vi "WhiteScreenTest_Startup.vi"() -> (0 "ErrorOut":errorcluster)   [LabVIEW 2018] (continued)
-51.99405193395278, -67.01264267414084, -53.44571979526376, -57.99170790064061, -81.70961030405843, -57.55954298568111, -65.02167716156492, -63.670039415871095, -66.27707836992371, -72.55910236513691, -72.7711109939143, -62.13879248220557, -81.54101193978573, -58.629597809474696, -56.28921520683527, -62.01138186186228, -61.61803085838006, -67.34927370509035, -71.65909904633395, -51.41437767083715, -80.31871825611697, -68.62589077386892, -56.503103976004134, -68.56520281728666, -68.07660380418503, -66.43496315022747, -80.55706592055753, -58.34547433203358, -80.86357761750227, -67.11611209017593, -67.39506376816462, -61.3536075715084, -57.86340014748689, -63.774368883554196, -65.72800124970155, -52.20213098851085, -59.70633504561058, -84.09135578340957, -93.10187122260785, -115.8843421262331, -59.4590004904725, -54.15581280534354, -64.41974754094588, -65.11772802657723, -59.72007368025384, -54.860367458875366, -64.71599198424335, -88.15700585273521, -67.79336517822267, -53.60791978937983, -63.288608307220095, -58.97631404304433, -56.56722195249055, -56.08704954963907, -53.87328284835936, -54.328629340092355, -55.41015013610399, -66.24988345447511, -63.81115391904144, -59.56325497844647, -56.94831717827518, -61.65160219622933, -64.17056469987938, -77.14151841475712, -65.6193156486078, -58.86248673523286, -60.1165495622408, -63.36871733225281, -60.84953671101233, -74.8582840465121, -59.88998847841493, -95.93625941689842, -59.88299394657023, -58.812327143828576, -60.07365977395545, -60.65812972265841, -55.29460982336834, -54.39350693136425, -64.44221359336854, -56.66420968725436, -57.849249090192934, -58.12466513592309, -57.45583386749336, -54.61500881558725, -61.345460649574996, -58.25358949545251, -54.81079112114542, -69.31075240072312, -75.37140100124691, -80.95747396257286, -65.41178936486318, -52.611019655802245, -65.58758224223078, -63.071696702033954, -108.10508856206985, -60.231868757101445, -73.66935735300541, -54.45286974455788, -65.5685924636773, -67.99482155268655, -61.14400427511112, -58.82484247502318, -60.60898321122287, -59.39233587194578, -63.81115391904144, -61.2240798652709, -73.46555302607382, -62.66606303410514, -59.16259174067152, -64.56672625582956, -56.53264364522695, -57.97450072113913, -57.74797307623616, -69.70157942586468, -66.1016740458054, -78.55011000645786, -69.9180460463688, -57.80973682485905, -52.29836944058602, -65.19040261658174, -54.23115847512327, -70.88024189200894, -52.42606516970066, -88.9193056485365, -84.95782085255706, -53.597020716062, -59.4256102722857, -58.68806374826783, -69.35757045363206, -51.922125139306594, -62.54072323990115, -69.50894243068942, -84.004540711267, -70.72744912841324, -64.00259486210794, -60.377994964097574, -70.54512838063863, -53.717597051139585, -55.80413177641689, -55.66574153199439, -61.19196937503859, -70.21106198010139, -71.59962582422565, -54.769672326943116, -66.36599807965678, -82.71277721205894, -52.74962062202692, -61.4436833506844, -85.00566633827245, -86.4525103194963, -70.3349775889819, -71.30766780674031, -64.72757074243842, -59.04654597071872, -63.24880327085554, -65.72800124970155, -49.792492705188714, -65.00973814322239, -51.33087211577806, -80.23084283247556, -54.61097220706987, -60.876641068095076, -67.42571235653492, -65.09362499882167, -58.53496442470185, -60.58262362643337, -96.55537745017114, -56.98701428601347, -53.28797453185026, -82.1980867315271, -59.027340759098955, -79.26102778332853, -65.3435997401024, -78.11942920258147, -64.15418040896233, -66.17549252828113, -52.62905623918589, -61.42724290107348, -77.7072560203516, -64.62386162425068, -57.423315192286346, -77.09935131389628, -60.27183207943016, -75.62058384231338, -57.708874914398926, -56.58703708992575, -62.92176524070543, -52.13798445576547, -58.60202729712321, -72.01150979498112, -59.50930474837666, -75.2665584276316, -70.90226945622248, -56.44429612900094, -51.53222748846188, -55.38386792788341, -64.08892165389514, -58.14797741957073, -90.74071668652113, -84.22306952305414, -59.67207429490822, -52.276196407765845, -68.53069558583377, -68.44496668642603, -58.11884590614199, -62.16093188737036, -62.62410087728153, -68.44496668642603, -58.39025269247278, -59.94612909219138, -73.32258465708762, -57.55954298568111, -53.4833218966046, -55.42771169707262, -65.04559986722944, -65.02167716156492, -64.87938036213663, -52.1099574921515, -59.95669213234839, -53.6662582435933, -67.198199716695, -55.663489389713824, -75.93213175750054, -66.78742748371917, -65.41178936486318, -58.20650719235265, -65.0815961571202, -78.00314899099467, -84.40154908991724, -54.75327403235176, -83.83323258754874, -74.69316809415548, -64.46473238305185, -69.01640908021349, -50.83910224754056, -60.7380559933847, -51.59980479701239, -55.42331829191223, -63.43936573152218, -61.32918753286523, -115.8843421262331, -58.48044138560088, -71.73095706023176, -72.63805754335351, -61.30888487978432, -56.00736133181352, -52.9460711732055, -62.294852163718495, -59.83417450278508, -52.545716476460804, -87.0271131916835, -56.06589110459543, -92.66575066808954, -78.74791082859372, -68.80143089608728, -53.00904327904521, -63.74817995109995, -70.04829243356986, -65.54964020199756, -61.12011136114078, -83.0197794113686, -66.44881586021592, -68.03562552743497, -60.98583086480918, -67.75357665166754, -62.79306219219861, -57.38282125288405, -61.47664901886427, -59.17232588661076, -65.31276396941814, -72.97421667524495, -60.27183207943016, -64.35823581751049, -51.88560352159029, -62.698827642682254, -58.31870730180095, -59.114068622547016, -80.1437650787519, -76.74822277376467, -65.02167716156492, -61.349533245687944, -59.1237536309416, -74.89165103667418, -62.21873461150245, -49.9438768204733, -55.64773918094529, -57.1591608304284, -50.85955205276931, -78.11942920258147, -68.8458224607262, -75.2665584276316, -71.68299196030429, -51.86133279390611, -61.59710827647664, -84.26737907065356, -64.36381152240443, -74.62790933908832, -57.46126437995087, -96.55537745017114, -71.37693164554997, -110.5159478725686, -76.87068826675005, -62.77414108152802, -60.81480040268996, -69.58553365591192, -53.578883066491635, -55.38824329854079, -66.51838106716721, -52.92573624243261, -60.08079476870609, -53.76182148597548, -60.989753580055, -82.34234508908514, -58.86248673523286, -67.13843005293714, -63.14509415266779, -70.78173902996198, -62.984354672270875, -61.98523100514074, -53.52467497348035, -64.19793419062762, -63.35866704322458, -59.322833066623296, -66.06164756214434, -65.43047096765142, -59.702903459095715, -54.41918572771261, -55.069738493302985, -88.0246865135197, -63.10098832784568, -51.225375139342894, -68.70448657082216, -55.57383453153566, -63.01338041302321, -59.41894615253175, -51.391268957464284, -80.0574706437699, -76.97395083542065, -57.65329538465085, -73.29424490235556, -59.43895241630013, -61.534612941440336, -73.07049131842601, -55.25352624879768, -73.96822887751696, -56.56474793571346, -69.64338106738398, -65.14189176731313, -71.87630832579441, -71.45837664659064, -49.74741788735506, -94.03851706113451, -58.806075595871924, -68.58250309248953, -82.78861159907069, -66.70876658826313, -68.462051285777, -57.05966921811025, -59.45565623385853, -53.25463195735258, -73.98341969620992, -70.82539325774144, -71.49349444053763, -69.13489894768142, -60.47790367814803, -59.15286746208921, -69.45189766398155, -62.727000937528324, -84.3118942317391, -56.6367547446168, -75.23186399560109, -52.1660935431082, -60.907711540600666, -56.26760663806902, -74.33961719286634, -65.93598771642783, -62.10788290425561, -74.33961719286634, -57.7647783360084, -54.58276340707521, -78.9754234684336, -80.52694658655275, -73.43678838683073, -75.67483280875109, -58.58369087867003, -64.79733832268226, -84.8628398786199, -61.85553547398538, -62.797798306834416, -49.456535410939274, -74.32385219342672, -54.37970830574462, -63.096100174873676, -56.06354304437077, -95.64106689530826, -70.88024189200894, -68.58250309248953, -78.45271830700355, -64.36381152240443, -78.16633883150865, -58.73757611624553, -67.97042221778648, -58.12175507978066, -57.321060647676155, -59.3459447625382, -59.11084245806395, -55.9144501939028, -72.93325006494365, -67.13843005293714, -63.135275318647835, -72.24962391387751, -59.28005851453177, -65.13584512355794, -66.50442761016166, -56.935452753657195, -70.55575774460704, -63.14018347940979, -64.94433782793823, -85.7535514055914, -69.52803298425346, -51.88864168471941, -64.22538199189958, -94.67404741663125, -58.07820983932687, -61.501447826297984, -72.40311518841392, -65.9031911032867, -65.74086912554111, -70.75998618617399, -58.743783169195815, -72.33886176668707, -68.57384905491571, -56.231700170696165, -76.95320920571854, -66.3043505986688, -55.827010394463606, -59.37242649088039, -61.47664901886427, -54.75327403235176, -57.20929627668493, -57.75357155903293, -64.70442718477156, -70.66270422572774, -59.448971216166406, -69.64338106738398, -62.35799390554727, -61.345460649574996, -60.17043287185472, -63.78486450823356, -81.24480659023706, -57.16705955462927, -62.085865451395556, -59.542988069499735, -59.23420591784562, -67.47958413870552, -57.64221801621441, -61.702180520776785, -65.52442862375423, -74.41883316736389, -66.1016740458054, -68.3093743230275, -72.79794457784413, -83.66493002506755, -62.78359697189443, -62.727000937528324, -62.79306219219861, -69.97794010149332, -106.18005458050143, -91.09605360575071, -80.0574706437699, -90.5678651632339, -84.17896369823202, -63.27366205646876, -70.90226945622248, -93.44248688497498, -61.71486687924905, -61.484908167028344, -86.4525103194963, -62.10347536914477, -65.84443828268391, -69.64338106738398, -92.55974958955161, -60.93108061427673, -61.88994986066991, -70.97976670400445, -72.63805754335351, -59.188571445108, -59.027340759098955, -90.23123413228441, -67.28855831253992, -61.52216258278157, -60.268192162862114, -70.7382825570067, -63.36871733225281, -56.32533800588815, -78.94987618302852, -75.11141218888855, -70.64121933432824, -62.916967541180576, -56.0494667395707, -61.72333378182871, -59.322833066623296, -59.130215739639986, -73.84756061980656, -64.70442718477156, -63.51053828904819, -65.09964508060068, -85.29786151567325, -56.38827489577944, -89.43797250218225, -73.3795165749292, -70.20080756971822, -64.09976733057331, -67.25834411433442, -67.4333898279331, -66.46268860305295, -71.37693164554997, -48.24420036050936, -68.10951292736854, -72.12356428124627, -52.92065923781558, -62.43979165363363, -65.06958237972034, -62.394262379750494, -72.63805754335351, -65.03363105719274, -72.35167806785861, -65.27589140640507, -55.767639102832625, -70.01807823536436, -70.82539325774144, -67.5804415173883, -65.72157377877431, -60.084364257119354, -69.7601330155891, -58.83110626891206, -108.65340922603647, -67.00529453130741, -60.876641068095076, -59.542988069499735, -63.75864694613728, -80.64799551131347, -58.30683477553303, -75.65671571177037, -83.45862099838286, -57.35860668386382, -56.33016467265663, -71.238900487172, -91.0059778265747, -68.86363676482424, -60.715151883817335, -76.29274197049554, -69.26416173119159, -71.10282728369415, -62.54072323990115, -71.63526549370167, -65.67670166221052, -72.61166688021697, -56.56474793571346, -87.95920503059935, -60.006140695445445, -59.4590004904725, -54.250573579908725, -59.80638882079618, -63.449500967541546, -64.64106880375215, -75.02629184336465, -72.71766795875487, -73.09817676332747, -66.84504327252878, -82.5257732396841, -57.87757211047214, -53.427865704868985, -62.35346997242876, -58.0003230785883, -56.33982529784368, -70.63049490615708, -82.16235857104732, -60.80324952832628, -64.9088519674983, -70.01807823536436, -77.75218818680568, -57.58152008578582, -61.26436971869881, -55.120674896161084, -60.5901475483877, -83.83323258754874, -59.472389187691185, -64.54396705179721, -69.19008414301271, -66.16202866642189, -62.52229287880461, -66.24309675451039, -88.15700585273521, -76.44872914721853, -75.87641233657254, -71.03550770917977, -64.15418040896233, -56.81282418633612, -56.76471348763396, -79.26102778332853, -65.02167716156492, -57.05966921811025, -68.6345919082523, -78.77292518435783, -80.80148678584987, -71.19332795490877, -60.41118238908704, -63.30857293461339, -60.21375850063715, -69.03454330111458, -63.790116629908674, -55.538205892623374, -66.25667495918356, -76.56740694948036, -73.05667850106471, -58.36634489193626, -60.07365977395545, -57.59528138494674, -70.20080756971822, -66.02178739399196, -78.72296152974505, -52.49055616889071, -57.614580428673754, -54.21178258487631, -63.08145064288444, -81.88122489871265, -60.96232819890859, -84.26737907065356, -77.18387168443718, -59.104393382190814, -58.209443076078706, -75.78425985079298, -83.17704522854666, -72.93325006494365, -55.656736133539106, -73.62531902011878, -56.77988028921224, -62.02011467994374, -68.38540906718583, -67.05685012564672, -59.22767340142021, -56.50556214385872, -63.32857919838175, -74.01387369004044, -95.07660997858827, -58.18012459360005, -64.13237812685045, -60.41857299037708, -63.98649471846863, -78.3084599494455, -88.9917059921967, -53.82854277503649, -53.27743277254765, -52.8599438452651, -66.94671114313334, -55.39700003123463, -72.08606716510013, -54.225341597734335, -67.7853942596087, -71.10282728369415, -59.98138455267408, -82.5628835374147, -55.95150673442901, -68.82804117667325, -54.39942670939845, -79.8310766559049, -56.953467782425754, -72.19900110510912, -60.253646291993284, -61.11216026246759, -73.18171575279334, -59.56663696332196, -56.38827489577944, -63.05221852275313, -71.03550770917977, -79.91534952583305, -65.98869664024195, -73.46555302607382, -74.5954456871255, -58.4412554709403, -77.91112910075469, -59.00179347369386, -85.15065146578425, -57.1119045772306, -71.97444728912444, -111.99471534415147, -72.17378952686579, -70.54512838063863, -66.18897531335372, -68.20892314340054, -66.04169677505735, -70.1701099435229, -103.86658696945702, -62.764694502724275, -68.54793368571038, -61.567893113587196, -68.97122293920182, -67.44107344868831, -67.18322235221623, -59.04654597071872, -63.24880327085554, -58.08400446348373, -72.53292772406871, -68.56520281728666, -61.18796311062453, -66.16875823527027, -85.9632428146347, -72.66452100841161, -63.99185843121669, -76.8092600952713, -65.80546869625675, -63.530970671639516, -69.87832342232358, -82.9421028736071, -66.1016740458054, -99.10426791904789, -73.81762923826997, -72.27503584926745, -58.32167773068364, -71.47006829946992, -68.42791245971216, -66.881229660213, -76.44872914721853, -81.57449539437292, -75.78425985079298, -72.65128015054688, -72.94688617242807, -75.58458755242262, -61.31700078551376, -55.772193102443445, -67.3188679744054, -62.5591890781343, -61.702180520776785, -71.13666506128303, -71.49349444053763, -72.08606716510013, -97.39007758963268, -67.80134272545996, -75.44193808375724, -66.8739814543525, -63.863949869585916, -66.40041864044619, -60.593911723440904, -85.00566633827245, -68.20892314340054, -71.40013117318102, -71.70694453204936, -84.3118942317391, -64.08350341031704, -73.3795165749292, -68.66947558305529, -64.90295039856406, -76.44872914721853, -64.87938036213663, -67.36451278692888, -76.2156893474037, -71.803357403892, -80.23084283247556, -68.66947558305529, -81.95073969565235, -72.50682430660166, -74.66048322437624, -65.04559986722944, -74.05973672560452, -72.66452100841161, -74.29239970623465, -72.49379918579547, -59.66181988452505, -69.47087492041769, -84.49204976113185, -67.52600197120663, -66.95401453138103, -79.42047189702586, -63.94369263965309, -83.66493002506755, -88.56528023385471, -78.92439675237901, -77.3768100315248, -88.56528023385471, -79.42047189702586, -82.05596561359027, -78.16633883150865, -75.54872582841557, -77.14151841475712, -77.77473343807586, -73.87758568344123, -66.04169677505735, -83.54061295051198, -74.57925496598259, -78.4769736928713, -70.69502205528289, -78.11942920258147, -65.03363105719274, -70.70581890504388, -82.78861159907069, -71.99913970945016, -70.74912823368484, -80.1437650787519, -71.92525230951662, -77.3984891367964, -74.02913701863835, -70.66270422572774, -70.53451078132562, -81.44125714141563, -77.5296027951205, -90.39807312011936, -70.09886187065311, -72.12356428124627, -92.45490701593633, -88.70532651670183, -68.49631203647937, -97.21722606634546, -104.95374904760712, -75.35384747393371, -75.60256881354482, -97.21722606634546, -79.20846326824847, -96.3968118565532, -72.3773621528131, -81.37532561040814, -71.02433356697281, -81.30984412748779, -67.42571235653492, -78.35630543516089, -81.40823473359166, -85.70183699463703, -71.803357403892, -89.21224444052623, -93.32759928426387, -89.13816685234738, -78.18987994761696, -96.88059503539597, -77.84268885802032, -108.65340922603647, -95.35468741981339, -71.82761278975974, -75.83944504612427, -103.86658696945702, -85.24854007026573, -79.97194556019917, -80.37775228857197, -90.74071668652113, -88.63504781409856, -73.02911239014207, -83.25665564394805, -89.90601654705961, -75.11141218888855, -100.20812799967334, -85.49772291133223, -71.25032752842785, -78.89898481698907, -89.74745095344164, -78.35630543516089, -76.2156893474037, -80.31871825611697, -76.62730100460487, -84.35661692346315, -86.1235752376158, -85.24854007026573, -86.90940619345022, -105.75362882215944, -102.58562032000998, -88.9193056485365, -81.50764494962365, -84.26737907065356, -80.55706592055753, -85.91038868644006, -79.85908543492619, -86.177620450987, -87.57543385565012, -77.57370861994258, -93.79564332914123, -100.93706080531254, -107.5864217084241, -76.48812550649035, -85.19947090956941, -96.24082467983021, -83.0197794113686, -86.67823838115231, -82.0912989868688, -72.81138956953345, -89.59146377671865, -79.05247609152548, -86.9680791592285, -89.59146377671865, -111.22686564943922, -95.35468741981339, -77.77473343807586, -84.004540711267, -82.34234508908514, -96.55537745017114, -80.92607295253859, -110.5159478725686, -75.80261966500962, -78.5991791671542, -85.19947090956941, -84.004540711267, -84.81569973462018, -86.90940619345022, -84.35661692346315, -81.30984412748779, -82.60013795316792, -95.78752775545891, -117.16530877568013, -84.768790105693, -84.72210874836932, -76.2156893474037, -91.37146965148088, -88.9917059921967, -108.10508856206985, -90.23123413228441, -89.43797250218225, -82.26994474542494, -86.79312598186345, -82.78861159907069, -108.65340922603647, -87.89416749334862, -87.08651276227181, -97.92814384321613, -86.4525103194963, -95.93625941689842, -80.55706592055753, -79.80314941638477, -95.07660997858827, -90.39807312011936, -95.93625941689842, -90.14889027905289, -105.34535444103992, -112.82941548361299, -87.26695068374008, -90.91673997376512, -91.75144011322664, -92.45490701593633, -85.85782417136002, -102.89018558294177, -95.93625941689842, -107.5864217084241, -102.29042779841981, -90.23123413228441, -82.26994474542494, -91.27878294010458, -82.71277721205894, -118.64407624726303, -82.23394845553418, -91.9472224187848, -89.43797250218225, -82.67508364686299, -109.23498122312157, -86.62130646331073, -98.89795889236316, -106.18005458050143, -86.79312598186345, -87.82956792263298, -99.3151115712011, -87.70165936100221, -99.10426791904789, -89.51441115362678, -112.82941548361299, -93.55876709656178, -115.8843421262331, -87.26695068374008, -87.51293852061383, -84.62942203699302, -94.54352839646018, -87.38915615802296, -88.0246865135197, -103.86658696945702, -94.28769990220098, -92.2485979892516, -93.79564332914123, -110.5159478725686, -88.42724907547671, -83.05885482181219, -87.14628242602967, -90.39807312011936, -91.84883181268097, -97.39007758963268, -101.45572765895832, -80.86357761750227, -101.19288929957173, -96.55537745017114, -81.74368849264914, -88.70532651670183, -86.62130646331073, -86.56471042894461, -93.44248688497498, -83.49952937594134, -93.32759928426387, -97.21722606634546, -101.19288929957173, -103.20473835328269, -84.8628398786199, -94.54352839646018, -110.5159478725686, -88.22385629748447, -95.93625941689842, -94.03851706113451, -99.97696018737543, -113.7437260384759, -86.177620450987, -89.06465691409912, -120.39308694158743, -91.75144011322664, -91.75144011322664, -93.67647409479505, -89.59146377671865, -113.7437260384759, -93.32759928426387, -97.92814384321613, -94.80636675584677, -86.34160735020279, -97.92814384321613, -92.0466326348168, -91.84883181268097, -125.29343715037459, -96.3968118565532, -86.90940619345022, -92.14708381444379, -91.55957371750958, -101.45572765895832, -95.93625941689842, -88.42724907547671, -100.44500423225278, -92.55974958955161, -94.54352839646018, -97.56610087687667, -87.38915615802296, -111.99471534415147, -93.32759928426387, -88.0246865135197, -100.20812799967334, -91.27878294010458, -91.27878294010458, -96.24082467983021, -90.14889027905289, -96.55537745017114, -91.9472224187848, -89.06465691409912, -117.16530877568013, -91.46506063773174, -93.79564332914123, -103.86658696945702, -88.84744763463866, -125.29343715037459, -93.32759928426387, -89.51441115362678, -109.23498122312157, -94.16229942372536, -92.88133277427832, -97.39007758963268, -92.0466326348168, -96.3968118565532, -93.32759928426387, -88.70532651670183, -129.1830639324562, -92.2485979892516, -97.21722606634546, -97.92814384321613, -90.91673997376512, -97.04743402323092, -100.68787796424607, -88.84744763463866, -105.34535444103992, -91.09605360575071, -94.28769990220098, -95.64106689530826, -90.06724723306866, -93.79564332914123, -92.14708381444379, -89.3621381151705, -125.29343715037459, -91.0059778265747, -89.90601654705961, -102.00404832292494, -88.29117587199889, -109.23498122312157, -97.39007758963268, -86.34160735020279, -103.52995593850753, -90.3142909281791, -99.10426791904789, -91.84883181268097, -90.5678651632339, -93.79564332914123, -94.54352839646018, -90.74071668652113, -107.09436513536431, -89.74745095344164, -95.49680853775021, -92.77293614072735, -90.06724723306866, -113.7437260384759, -91.84883181268097, -89.43797250218225, -135.8324248355678, -96.88059503539597, -94.03851706113451, -100.44500423225278, -89.82640613165822, -96.3968118565532, -96.88059503539597, -91.37146965148088, -125.29343715037459, -90.91673997376512, -97.04743402323092, -113.7437260384759]
  out "NoiseFloor 4":dbl[](graph)=[-inf, -inf, -inf, -inf, -inf, -inf, -inf, -inf, -inf, -inf, -inf, -inf, -inf, -inf, -inf, -inf, -inf, -inf, -inf, -inf, -inf, -inf, -inf, -inf, -inf, -inf, -inf, -inf, -inf, -inf, -inf, -inf, -inf, -inf, -inf, -inf, -inf, -inf, -inf, -inf, -inf, -inf, -inf, -inf, -inf, -inf, -inf, -inf, -inf, -inf, -inf, -inf, -inf, -inf, -inf, -inf, -inf, -inf, -inf, -inf, -inf, -inf, -inf, -inf, -inf, -inf, -inf, -inf, -inf, -inf, -inf, -inf, -inf, -inf, -inf, -inf, -inf, -inf, -inf, -inf, -inf, -inf, -inf, -inf, -inf, -inf, -inf, -inf, -inf, -inf, -inf, -inf, -inf, -inf, -inf, -inf, -inf, -inf, -inf, -inf, -inf, -inf, -inf, -inf, -inf, -inf, -inf, -inf, -inf, -inf, -inf, -inf, -inf, -inf, -inf, -inf, -inf, -inf, -inf, -inf, -inf, -inf, -inf, -inf, -inf, -inf, -inf, -inf, -inf, -inf, -inf, -inf, -inf, -inf, -inf, -inf, -inf, -inf, -inf, -inf, -inf, -inf, -inf, -inf, -inf, -inf, -inf, -inf, -inf, -inf, -inf, -inf, -inf, -inf, -inf, -inf, -inf, -inf, -inf, -inf, -inf, -inf, -inf, -inf, -inf, -inf, -inf, -inf, -inf, -inf, -inf, -inf, -inf, -inf, -inf, -inf, -inf, -inf, -inf, -inf, -inf, -inf, -inf, -inf, -inf, -inf, -inf, -inf, -inf, -inf, -inf, -inf, -inf, -inf, -inf, -inf, -inf, -inf, -inf, -inf, -inf, -inf, -inf, -inf, -inf, -inf, -inf, -inf, -inf, -inf, -inf, -inf, -inf, -inf, -inf, -inf, -inf, -inf, -inf, -inf, -inf, -inf, -inf, -inf, -inf, -inf, -inf, -inf, -inf, -inf, -inf, -inf, -inf, -inf, -inf, -inf, -inf, -inf, -inf, -inf, -inf, -inf, -inf, -inf, -inf, -inf, -inf, -inf, -inf, -inf, -inf, -inf, -inf, -inf, -inf, -inf, -inf, -inf, -inf, -inf, -inf, -inf, -inf, -inf, -inf, -inf, -inf, -inf, -inf, -inf, -inf, -inf, -inf, -inf, -inf, -inf, -inf, -inf, -inf, -inf, -inf, -inf, -inf, -inf, -inf, -inf, -inf, -inf, -inf, -inf, -inf, -inf, -inf, -inf, -inf, -inf, -inf, -inf, -inf, -inf, -inf, -inf, -inf, -inf, -inf, -inf, -inf, -inf, -inf, -inf, -inf, -inf, -inf, -inf, -inf, -inf, -inf, -inf, -inf, -inf, -inf, -inf, -inf, -inf, -inf, -inf, -inf, -inf, -inf, -inf, -inf, -inf, -inf, -inf, -inf, -inf, -inf, -inf, -inf, -inf, -inf, -inf, -inf, -inf, -inf, -inf, -inf, -inf, -inf, -inf, -inf, -inf, -inf, -inf, -inf, -inf, -inf, -inf, -inf, -inf, -inf, -inf, -inf, -inf, -inf, -inf, -inf, -inf, -inf, -inf, -inf, -inf, -inf, -inf, -inf, -inf, -inf, -inf, -inf, -inf, -inf, -inf, -inf, -inf, -inf, -inf, -inf, -inf, -inf, -inf, -inf, -inf, -inf, -inf, -inf, -inf, -inf, -inf, -inf, -inf, -inf, -inf, -inf, -inf, -inf, -inf, -inf, -inf, -inf, -inf, -inf, -inf, -inf, -inf, -inf, -inf, -inf, -inf, -inf, -inf, -inf, -inf, -inf, -inf, -inf, -inf, -inf, -inf, -inf, -inf, -inf, -inf, -inf, -inf, -inf, -inf, -inf, -inf, -inf, -inf, -inf, -inf, -inf, -inf, -inf, -inf, -inf, -inf, -inf, -inf, -inf, -inf, -inf, -inf, -inf, -inf, -inf, -inf, -inf, -inf, -inf, -inf, -inf, -inf, -inf, -inf, -inf, -inf, -inf, -inf, -inf, -inf, -inf, -inf, -inf, -inf, -inf, -inf, -inf, -inf, -inf, -inf, -inf, -inf, -inf, -inf, -inf, -inf, -inf, -inf, -inf, -inf, -inf, -inf, -inf, -inf, -inf, -inf, -inf, -inf, -inf, -inf, -inf, -inf, -inf, -inf, -inf, -inf, -inf, -inf, -inf, -inf, -inf, -inf, -inf, -inf, -inf, -inf, -inf, -inf, -inf, -inf, -inf, -inf, -inf, -inf, -inf, -inf, -inf, -inf, -inf, -inf, -inf, -inf, -inf, -inf, -inf, -inf, -inf, -inf, -inf, -inf, -inf, -inf, -inf, -inf, -inf, -inf, -inf, -inf, -inf, -inf, -inf, -inf, -inf, -inf, -inf, -inf, -inf, -inf, -inf, -inf, -inf, -inf, -inf, -inf, -inf, -inf, -inf, -inf, -inf, -inf, -inf, -inf, -inf, -inf, -inf, -inf, -inf, -inf, -inf, -inf, -inf, -inf, -inf, -inf, -inf, -inf, -inf, -inf, -inf, -inf, -inf, -inf, -inf, -inf, -inf, -inf, -inf, -inf, -inf, -inf, -inf, -inf, -inf, -inf, -inf, -inf, -inf, -inf, -inf, -inf, -inf, -inf, -inf, -inf, -inf, -inf, -inf, -inf, -inf, -inf, -inf, -inf, -inf, -inf, -inf, -inf, -inf, -inf, -inf, -inf, -inf, -inf, -inf, -inf, -inf, -inf, -inf, -inf, -inf, -inf, -inf, -inf, -inf, -inf, -inf, -inf, -inf, -inf, -inf, -inf, -inf, -inf, -inf, -inf, -inf, -inf, -inf, -inf, -inf, -inf, -inf, -inf, -inf, -inf, -inf, -inf, -inf, -inf, -inf, -inf, -inf, -inf, -inf, -inf, -inf, -inf, -inf, -inf, -inf, -inf, -inf, -inf, -inf, -inf, -inf, -inf, -inf, -inf, -inf, -inf, -inf, -inf, -inf, -inf, -inf, -inf, -inf, -inf, -inf, -inf, -inf, -inf, -inf, -inf, -inf, -inf, -inf, -inf, -inf, -inf, -inf, -inf, -inf, -inf, -inf, -inf, -inf, -inf, -inf, -inf, -inf, -inf, -inf, -inf, -inf, -inf, -inf, -inf, -inf, -inf, -inf, -inf, -inf, -inf, -inf, -inf, -inf, -inf, -inf, -inf, -inf, -inf, -inf, -inf, -inf, -inf, -inf, -inf, -inf, -inf, -inf, -inf, -inf, -inf, -inf, -inf, -inf, -inf, -inf, -inf, -inf, -inf, -inf, -inf, -inf, -inf, -inf, -inf, -inf, -inf, -inf, -inf, -inf, -inf, -inf, -inf, -inf, -inf, -inf, -inf, -inf, -inf, -inf, -inf, -inf, -inf, -inf, -inf, -inf, -inf, -inf, -inf, -inf, -inf, -inf, -inf, -inf, -inf, -inf, -inf, -inf, -inf, -inf, -inf, -inf, -inf, -inf, -inf, -inf, -inf, -inf, -inf, -inf, -inf, -inf, -inf, -inf, -inf, -inf, -inf, -inf, -inf, -inf, -inf, -inf, -inf, -inf, -inf, -inf, -inf, -inf, -inf, -inf, -inf, -inf, -inf, -inf, -inf, -inf, -inf, -inf, -inf, -inf, -inf, -inf, -inf, -inf, -inf, -inf, -inf, -inf, -inf, -inf, -inf, -inf, -inf, -inf, -inf, -inf, -inf, -inf, -inf, -inf, -inf, -inf, -inf, -inf, -inf, -inf, -inf, -inf, -inf, -inf, -inf, -inf, -inf, -inf, -inf, -inf, -inf, -inf, -inf, -inf, -inf, -inf, -inf, -inf, -inf, -inf, -inf, -inf, -inf, -inf, -inf, -inf, -inf, -inf, -inf, -inf, -inf, -inf, -inf, -inf, -inf, -inf, -inf, -inf, -inf, -inf, -inf, -inf, -inf, -inf, -inf, -inf, -inf, -inf, -inf, -inf, -inf, -inf, -inf, -inf, -inf, -inf, -inf, -inf, -inf, -inf, -inf, -inf, -inf, -inf, -inf, -inf, -inf, -inf, -inf, -inf, -inf, -inf, -inf, -inf, -inf, -inf, -inf, -inf, -inf, -inf, -inf, -inf, -inf, -inf, -inf, -inf, -inf, -inf, -inf, -inf, -inf, -inf, -inf, -inf, -inf, -inf, -inf, -inf, -inf, -inf, -inf, -inf, -inf, -inf, -inf, -inf, -inf, -inf, -inf, -inf, -inf, -inf, -inf, -inf, -inf, -inf, -inf, -inf, -inf, -inf, -inf, -inf, -inf, -inf, -inf, -inf, -inf, -inf, -inf, -inf, -inf, -inf, -inf, -inf, -inf, -inf, -inf, -inf, -inf, -inf, -inf, -inf, -inf, -inf, -inf, -inf, -inf, -inf, -inf, -inf, -inf, -inf, -inf, -inf, -inf, -inf, -inf, -inf, -inf, -inf, -inf, -inf, -inf, -inf, -inf, -inf, -inf, -inf, -inf, -inf, -inf, -inf, -inf, -inf, -inf, -inf, -inf, -inf, -inf, -inf, -inf, -inf, -inf, -inf, -inf, -inf, -inf, -inf, -inf, -inf, -inf, -inf, -inf, -inf, -inf, -inf, -inf, -inf, -inf, -inf, -inf, -inf, -inf, -inf, -inf, -inf, -inf, -inf, -inf, -inf, -inf, -inf, -inf, -inf, -inf, -inf, -inf, -inf, -inf, -inf, -inf, -inf, -inf, -inf, -inf, -inf, -inf, -inf, -inf, -inf, -inf, -inf, -inf, -inf, -inf, -inf, -inf, -inf, -inf, -inf, -inf, -inf, -inf, -inf, -inf, -inf, -inf, -inf, -inf, -inf, -inf, -inf, -inf, -inf, -inf, -inf, -inf, -inf, -inf, -inf, -inf, -inf, -inf, -inf, -inf, -inf, -inf, -inf, -inf, -inf, -inf, -inf, -inf, -inf, -inf, -inf, -inf, -inf, -inf, -inf, -inf, -inf, -inf, -inf, -inf, -inf, -inf, -inf, -inf, -inf, -inf, -inf, -inf, -inf, -inf, -inf, -inf, -inf, -inf, -inf, -inf, -inf, -inf, -inf, -inf, -inf, -inf, -inf, -inf, -inf, -inf, -inf, -inf, -inf, -inf, -inf, -inf, -inf, -inf, -inf, -inf, -inf, -inf, -inf, -inf, -inf, -inf, -inf, -inf, -inf, -inf, -inf, -inf, -inf, -inf, -inf, -inf, -inf, -inf, -inf, -inf, -inf, -inf, -inf, -inf, -inf, -inf, -inf, -inf, -inf, -inf, -inf, -inf, -inf, -inf, -inf, -inf, -inf, -inf, -inf, -inf, -inf, -inf, -inf, -inf, -inf, -inf, -inf, -inf, -inf, -inf, -inf, -inf, -inf, -inf, -inf, -inf, -inf, -inf, -inf, -inf, -inf, -inf, -inf, -inf, -inf, -inf, -inf, -inf, -inf, -inf, -inf, -inf, -inf, -inf, -inf, -inf, -inf, -inf, -inf, -inf, -inf, -inf, -inf, -inf, -inf, -inf, -inf, -inf, -inf, -inf, -inf, -inf, -inf, -inf, -inf, -inf, -inf, -inf, -inf, -inf, -inf, -inf, -inf, -inf, -inf, -inf, -inf, -inf, -inf, -inf, -inf, -inf, -inf, -inf, -inf, -inf, -inf, -inf, -inf, -inf, -inf, -inf, -inf, -inf, -inf, -inf, -inf, -inf, -inf, -inf, -inf, -inf, -inf, -inf, -inf, -inf, -inf, -inf, -inf, -inf, -inf, -inf, -inf, -inf, -inf, -inf, -inf, -inf, -inf, -inf, -inf, -inf, -inf, -inf, -inf, -inf, -inf, -inf, -inf, -inf, -inf, -inf, -inf, -inf, -inf, -inf, -inf, -inf, -inf, -inf, -inf, -inf, -inf, -inf, -inf, -inf, -inf, -inf, -inf, -inf, -inf, -inf, -inf, -inf, -inf, -inf, -inf, -inf, -inf, -inf, -inf, -inf, -inf, -inf, -inf, -inf, -inf, -inf, -inf, -inf, -inf, -inf, -inf, -inf, -inf, -inf, -inf, -inf, -inf, -inf, -inf, -inf, -inf, -inf, -inf, -inf, -inf, -inf, -inf, -inf, -inf, -inf, -inf, -inf, -inf, -inf, -inf, -inf, -inf, -inf, -inf, -inf, -inf, -inf, -inf, -inf, -inf, -inf, -inf, -inf, -inf, -inf, -inf, -inf, -inf, -inf, -inf, -inf, -inf, -inf, -inf, -inf, -inf, -inf, -inf, -inf, -inf, -inf, -inf, -inf, -inf, -inf, -inf, -inf, -inf, -inf, -inf, -inf, -inf, -inf, -inf, -inf, -inf, -inf, -inf, -inf, -inf, -inf, -inf, -inf, -inf, -inf, -inf, -inf, -inf, -inf, -inf, -inf, -inf, -inf, -inf, -inf, -inf, -inf, -inf, -inf, -inf, -inf, -inf, -inf, -inf, -inf, -inf, -inf, -inf, -inf, -inf, -inf, -inf, -inf, -inf, -inf, -inf, -inf, -inf, -inf, -inf, -inf, -inf, -inf, -inf, -inf, -inf, -inf, -inf, -inf, -inf, -inf, -inf, -inf, -inf, -inf, -inf, -inf, -inf, -inf, -inf, -inf, -inf, -inf, -inf, -inf, -inf, -inf, -inf, -inf, -inf, -inf, -inf, -inf, -inf, -inf, -inf, -inf, -inf, -inf, -inf, -inf, -inf, -inf, -inf, -inf, -inf, -inf, -inf, -inf, -inf, -inf, -inf, -inf, -inf, -inf, -inf, -inf, -inf, -inf, -inf, -inf, -inf, -inf, -inf, -inf, -inf, -inf, -inf, -inf, -inf, -inf, -inf, -inf, -inf, -inf, -inf, -inf, -inf, -inf, -inf, -inf, -inf, -inf, -inf, -inf, -inf, -inf, -inf, -inf, -inf, -inf, -inf, -inf, -inf, -inf, -inf, -inf, -inf, -inf, -inf, -inf, -inf, -inf, -inf, -inf, -inf, -inf, -inf, -inf, -inf, -inf, -inf, -inf, -inf, -inf, -inf, -inf, -inf, -inf, -inf, -inf, -inf, -inf, -inf, -inf, -inf, -inf, -inf, -inf, -inf, -inf, -inf, -inf, -inf, -inf, -inf, -inf, -inf, -inf, -inf, -inf, -inf, -inf, -inf, -inf, -inf, -inf, -inf, -inf, -inf, -inf, -inf, -inf, -inf, -inf, -inf, -inf, -inf, -inf, -inf, -inf, -inf, -inf, -inf, -inf, -inf, -inf, -inf, -inf, -inf, -inf, -inf, -inf, -inf, -inf, -inf, -inf, -inf, -inf, -inf, -inf, -inf, -inf, -inf, -inf, -inf, -inf, -inf, -inf, -inf, -inf, -inf, -inf, -inf, -inf, -inf, -inf, -inf, -inf, -inf, -inf, -inf, -inf, -inf, -inf, -inf, -inf, -inf, -inf, -inf, -inf, -inf, -inf, -inf, -inf, -inf, -inf, -inf, -inf, -inf, -inf, -inf, -inf, -inf, -inf, -inf, -inf, -inf, -inf, -inf, -inf, -inf, -inf, -inf, -inf, -inf, -inf, -inf, -inf, -inf, -inf, -inf, -inf, -inf, -inf, -inf, -inf, -inf, -inf, -inf, -inf, -inf, -inf, -inf, -inf, -inf, -inf, -inf, -inf, -inf, -inf, -inf, -inf, -inf, -inf, -inf, -inf, -inf, -inf, -inf, -inf, -inf, -inf, -inf, -inf, -inf, -inf, -inf, -inf, -inf, -inf, -inf, -inf, -inf, -inf, -inf, -inf, -inf, -inf, -inf, -inf, -inf, -inf, -inf, -inf, -inf, -inf, -inf, -inf, -inf, -inf, -inf, -inf, -inf, -inf, -inf, -inf, -inf, -inf, -inf, -inf, -inf, -inf, -inf, -inf, -inf, -inf, -inf, -inf, -inf, -inf, -inf, -inf, -inf, -inf, -inf, -inf, -inf, -inf, -inf, -inf, -inf, -inf, -inf, -inf, -inf, -inf, -inf, -inf, -inf, -inf, -inf, -inf, -inf, -inf, -inf, -inf, -inf, -inf, -inf, -inf, -inf, -inf, -inf, -inf, -inf, -inf, -inf, -inf, -inf, -inf, -inf, -inf, -inf, -inf, -inf, -inf, -inf, -inf, -inf, -inf, -inf, -inf, -inf, -inf, -inf, -inf, -inf, -inf, -inf, -inf, -inf, -inf, -inf, -inf, -inf, -inf, -inf, -inf, -inf, -inf, -inf, -inf, -inf, -inf, -inf, -inf, -inf, -inf, -inf, -inf, -inf, -inf, -inf, -inf, -inf, -inf, -inf, -inf, -inf, -inf, -inf, -inf, -inf, -inf, -inf, -inf, -inf, -inf, -inf, -inf, -inf, -inf, -inf, -inf, -inf, -inf, -inf, -inf, -inf, -inf, -inf, -inf, -inf, -inf, -inf, -inf, -inf, -inf, -inf, -inf, -inf, -inf, -inf, -inf, -inf, -inf, -inf, -inf, -inf, -inf, -inf, -inf, -inf, -inf, -inf, -inf, -inf, -inf, -inf, -inf, -inf, -inf, -inf, -inf, -inf, -inf, -inf, -inf, -inf, -inf, -inf, -inf, -inf, -inf, -inf, -inf, -inf, -inf, -inf, -inf, -inf, -inf, -inf, -inf, -inf, -inf, -inf, -inf, -inf, -inf, -inf, -inf, -inf, -inf, -inf, -inf, -inf, -inf, -inf, -inf, -inf, -inf, -inf, -inf, -inf, -inf, -inf, -inf, -inf, -inf, -inf, -inf, -inf, -inf, -inf, -inf, -inf, -inf, -inf, -inf, -inf, -inf, -inf, -inf, -inf, -inf, -inf, -inf, -inf, -inf, -inf, -inf, -inf, -inf, -inf, -inf, -inf, -inf, -inf, -inf, -inf, -inf, -inf, -inf, -inf, -inf, -inf, -inf, -inf, -inf, -inf, -inf, -inf, -inf, -inf, -inf, -inf, -inf, -inf, -inf, -inf, -inf, -inf, -inf, -inf, -inf, -inf, -inf, -inf, -inf, -inf, -inf, -inf, -inf, -inf, -inf, -inf, -inf, -inf, -inf, -inf, -inf, -inf, -inf, -inf, -inf, -inf, -inf, -inf, -inf, -inf, -inf, -inf, -inf, -inf, -inf, -inf, -inf, -inf, -inf, -inf, -inf, -inf, -inf, -inf, -inf, -inf, -inf, -inf, -inf, -inf, -inf, -inf, -inf, -inf, -inf, -inf, -inf, -inf, -inf, -inf, -inf, -inf, -inf, -inf, -inf, -inf, -inf, -inf, -inf, -inf, -inf, -inf, -inf, -inf, -inf, -inf, -inf, -inf, -inf, -inf, -inf, -inf, -inf, -inf, -inf, -inf, -inf, -inf, -inf, -inf, -inf, -inf, -inf, -inf, -inf, -inf, -inf, -inf, -inf, -inf, -inf, -inf, -inf, -inf, -inf, -inf, -inf, -inf, -inf, -inf, -inf, -inf, -inf, -inf, -inf, -inf, -inf, -inf, -inf, -inf, -inf, -inf, -inf, -inf, -inf, -inf, -inf, -inf, -inf, -inf, -inf, -inf, -inf, -inf, -inf, -inf, -inf, -inf, -inf, -inf, -inf, -inf, -inf, -inf, -inf, -inf, -inf, -inf, -inf, -inf, -inf, -inf, -inf, -inf, -inf, -inf, -inf, -inf, -inf, -inf, -inf, -inf, -inf, -inf, -inf, -inf, -inf, -inf, -inf, -inf, -inf, -inf, -inf, -inf, -inf, -inf, -inf, -inf, -inf, -inf, -inf, -inf, -inf, -inf, -inf, -inf, -inf, -inf, -inf, -inf, -inf, -inf, -inf, -inf, -inf, -inf, -inf, -inf, -inf, -inf, -inf, -inf, -inf, -inf, -inf, -inf, -inf, -inf, -inf, -inf, -inf, -inf, -inf, -inf, -inf, -inf, -inf, -inf, -inf, -inf, -inf, -inf, -inf, -inf, -inf, -inf, -inf, -inf, -inf, -inf, -inf, -inf, -inf, -inf, -inf, -inf, -inf, -inf, -inf, -inf, -inf, -inf, -inf, -inf, -inf, -inf, -inf, -inf, -inf, -inf, -inf, -inf, -inf, -inf, -inf, -inf, -inf, -inf, -inf, -inf, -inf, -inf, -inf, -inf, -inf, -inf, -inf, -inf, -inf, -inf, -inf, -inf, -inf, -inf, -inf, -inf, -inf, -inf, -inf, -inf, -inf, -inf, -inf, -inf, -inf, -inf, -inf, -inf, -inf, -inf, -inf, -inf, -inf, -inf, -inf, -inf, -inf, -inf, -inf, -inf, -inf, -inf, -inf, -inf, -inf, -inf, -inf, -inf, -inf, -inf, -inf, -inf, -inf, -inf, -inf, -inf, -inf, -inf, -inf, -inf, -inf, -inf, -inf, -inf, -inf, -inf, -inf, -inf, -inf, -inf, -inf, -inf, -inf, -inf, -inf, -inf, -inf, -inf, -inf, -inf, -inf, -inf, -inf, -inf, -inf, -inf, -inf, -inf, -inf, -inf, -inf, -inf, -inf, -inf, -inf, -inf, -inf, -inf, -inf, -inf, -inf, -inf, -inf, -inf, -inf, -inf, -inf, -inf, -inf, -inf, -inf, -inf, -inf, -inf, -inf, -inf, -inf, -inf, -inf, -inf, -inf, -inf, -inf, -inf, -inf, -inf, -inf, -inf, -inf, -inf, -inf, -inf, -inf, -inf, -inf, -inf, -inf, -inf, -inf, -inf, -inf, -inf, -inf, -inf, -inf, -inf, -inf, -inf, -inf, -inf, -inf, -inf, -inf, -inf, -inf, -inf, -inf, -inf, -inf, -inf, -inf, -inf, -inf, -inf, -inf, -inf, -inf, -inf, -inf, -inf, -inf, -inf, -inf, -inf, -inf, -inf, -inf, -inf, -inf, -inf, -inf, -inf, -inf, -inf, -inf, -inf, -inf, -inf, -inf, -inf, -inf, -inf, -inf, -inf, -inf, -inf, -inf, -inf, -inf, -inf, -inf, -inf, -inf, -inf, -inf, -inf, -inf, -inf, -inf, -inf, -inf, -inf, -inf, -inf, -inf, -inf, -inf, -inf, -inf, -inf, -inf, -inf, -inf, -inf, -inf, -inf, -inf, -inf, -inf, -inf, -inf, -inf, -inf, -inf, -inf, -inf, -inf, -inf, -inf, -inf, -inf, -inf, -inf, -inf, -inf, -inf, -inf, -inf, -inf, -inf, -inf, -inf, -inf, -inf, -inf, -inf, -inf, -inf, -inf, -inf, -inf, -inf, -inf, -inf, -inf, -inf, -inf, -inf, -inf, -inf, -inf, -inf, -inf, -inf, -inf, -inf, -inf, -inf, -inf, -inf, -inf, -inf, -inf, -inf, -inf, -inf, -inf, -inf, -inf, -inf, -inf, -inf, -inf, -inf, -inf, -inf, -inf, -inf, -inf, -inf, -inf, -inf, -inf, -inf, -inf, -inf, -inf, -inf, -inf, -inf, -inf, -inf, -inf, -inf, -inf, -inf, -inf, -inf, -inf, -inf, -inf, -inf, -inf, -inf, -inf, -inf, -inf, -inf, -inf, -inf, -inf, -inf, -inf, -inf, -inf, -inf, -inf, -inf, -inf, -inf, -inf, -inf, -inf, -inf, -inf, -inf, -inf, -inf, -inf, -inf, -inf, -inf, -inf, -inf, -inf, -inf, -inf, -inf, -inf, -inf, -inf, -inf, -inf, -inf, -inf, -inf, -inf, -inf, -inf, -inf, -inf, -inf, -inf, -inf, -inf, -inf, -inf, -inf, -inf, -inf, -inf, -inf, -inf, -inf, -inf, -inf, -inf, -inf, -inf, -inf, -inf, -inf, -inf, -inf, -inf, -inf, -inf, -inf, -inf, -inf, -inf, -inf, -inf, -inf, -inf, -inf, -inf, -inf, -inf, -inf, -inf, -inf, -inf, -inf, -inf, -inf, -inf, -inf, -inf, -inf, -inf, -inf, -inf, -inf, -inf, -inf, -inf, -inf, -inf, -inf, -inf, -inf, -inf, -inf, -inf, -inf, -inf, -inf, -inf, -inf, -inf, -inf, -inf, -inf, -inf, -inf, -inf, -inf, -inf, -inf, -inf, -inf, -inf, -inf, -inf, -inf, -inf, -inf, -inf, -inf, -inf, -inf, -inf, -inf, -inf, -inf, -inf, -inf, -inf, -inf, -inf, -inf, -inf, -inf, -inf, -inf, -inf, -inf, -inf, -inf, -inf, -inf, -inf, -inf, -inf, -inf, -inf, -inf, -inf, -inf, -inf, -inf, -inf, -inf, -inf, -inf, -inf, -inf, -inf, -inf, -inf, -inf, -inf, -inf, -inf, -inf, -inf, -inf, -inf, -inf, -inf, -inf, -inf, -inf, -inf, -inf, -inf, -inf, -inf, -inf, -inf, -inf, -inf, -inf, -inf, -inf, -inf, -inf, -inf, -inf, -inf, -inf, -inf, -inf, -inf, -inf, -inf, -inf, -inf, -inf, -inf, -inf, -inf, -inf, -inf, -inf, -inf, -inf, -inf, -inf, -inf, -inf, -inf, -inf, -inf, -inf, -inf, -inf, -inf, -inf, -inf, -inf, -inf, -inf, -inf, -inf, -inf, -inf, -inf, -inf, -inf, -inf, -inf, -inf, -inf, -inf, -inf, -inf, -inf, -inf, -inf, -inf, -inf, -inf, -inf, -inf, -inf, -inf, -inf, -inf, -inf, -inf, -inf, -inf, -inf, -inf, -inf, -inf, -inf, -inf, -inf, -inf, -inf, -inf, -inf, -inf, -inf, -inf, -inf, -inf, -inf, -inf, -inf, -inf, -inf, -inf, -inf, -inf, -inf, -inf, -inf, -inf, -inf, -inf, -inf, -inf, -inf, -inf, -inf, -inf, -inf, -inf, -inf, -inf, -inf, -inf, -inf, -inf, -inf, -inf, -inf, -inf, -inf, -inf, -inf, -inf, -inf, -inf, -inf, -inf, -inf, -inf, -inf, -inf, -inf, -inf, -inf, -inf, -inf, -inf, -inf, -inf, -inf, -inf, -inf, -inf, -inf, -inf, -inf, -inf, -inf, -inf, -inf, -inf, -inf, -inf, -inf, -inf, -inf, -inf, -inf, -inf, -inf, -inf, -inf, -inf, -inf, -inf, -inf, -inf, -inf, -inf, -inf, -inf, -inf, -inf, -inf, -inf, -inf, -inf, -inf, -inf, -inf, -inf, -inf, -inf, -inf, -inf, -inf, -inf, -inf, -inf, -inf, -inf, -inf, -inf, -inf, -inf, -inf, -inf, -inf, -inf, -inf, -inf, -inf, -inf, -inf, -inf, -inf, -inf, -inf, -inf, -inf, -inf, -inf, -inf, -inf, -inf, -inf, -inf, -inf, -inf, -inf, -inf, -inf, -inf, -inf, -inf, -inf, -inf, -inf, -inf, -inf, -inf, -inf, -inf, -inf, -inf, -inf, -inf, -inf, -inf, -inf, -inf, -inf, -inf, -inf, -inf, -inf, -inf, -inf, -inf, -inf, -inf, -inf, -inf, -inf, -inf, -inf, -inf, -inf, -inf, -inf, -inf, -inf, -inf, -inf, -inf, -inf, -inf, -inf, -inf, -inf, -inf, -inf, -inf, -inf, -inf, -inf, -inf, -inf, -inf, -inf, -inf, -inf, -inf, -inf, -inf, -inf, -inf, -inf, -inf, -inf, -inf, -inf, -inf, -inf, -inf, -inf, -inf, -inf, -inf, -inf, -inf, -inf, -inf, -inf, -inf, -inf, -inf, -inf, -inf, -inf, -inf, -inf, -inf, -inf, -inf, -inf, -inf, -inf, -inf, -inf, -inf, -inf, -inf, -inf, -inf, -inf, -inf, -inf, -inf, -inf, -inf, -inf, -inf, -inf, -inf, -inf, -inf, -inf, -inf, -inf, -inf, -inf, -inf, -inf, -inf, -inf, -inf, -inf, -inf, -inf, -inf, -inf, -inf, -inf, -inf, -inf, -inf, -inf, -inf, -inf, -inf, -inf, -inf, -inf, -inf, -inf, -inf, -inf, -inf, -inf, -inf, -inf, -inf, -inf, -inf, -inf, -inf, -inf, -inf, -inf, -inf, -inf, -inf, -inf, -inf, -inf, -inf, -inf, -inf, -inf, -inf, -inf, -inf, -inf, -inf, -inf, -inf, -inf, -inf, -inf, -inf, -inf, -inf, -inf, -inf, -inf, -inf, -inf, -inf, -inf, -inf, -inf, -inf, -inf, -inf, -inf, -inf, -inf, -inf, -inf, -inf, -inf, -inf, -inf, -inf, -inf, -inf, -inf, -inf, -inf, -inf, -inf, -inf, -inf, -inf, -inf, -inf, -inf, -inf, -inf, -inf, -inf, -inf, -inf, -inf, -inf, -inf, -inf, -inf, -inf, -inf, -inf, -inf, -inf, -inf, -inf, -inf, -inf, -inf, -inf, -inf, -inf, -inf, -inf, -inf, -inf, -inf, -inf, -inf, -inf, -inf, -inf, -inf, -inf, 
